vi "Instantiate.vi"(0 "scripts manager in":refnum<class "scripts manager.lvclass">, 5 "Output Terminal":refnum<class "Output Terminal.lvclass">, 7 "RT Variables":refnum<class "RT Variables.lvclass">, 9 "Function Directory[]":path[](array[path]), 11 "error in (no error)":errorcluster) -> (4 "scripts manager out":refnum<class "scripts manager.lvclass">, 15 "error out":errorcluster)   [LabVIEW 2019, in "LSL.lvlib" / "scripts manager.lvclass"]
uses:
  scripts manager.lvclass
  output terminal/Base/Output Terminal.lvclass
  variables/RT Variables/RT Variables.lvclass
  scripts manager.lvclass/scripts manager.ctl
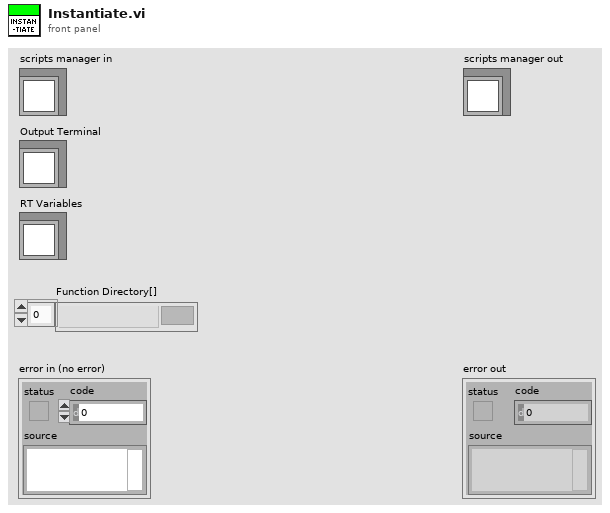
[diagram p1: front panel]
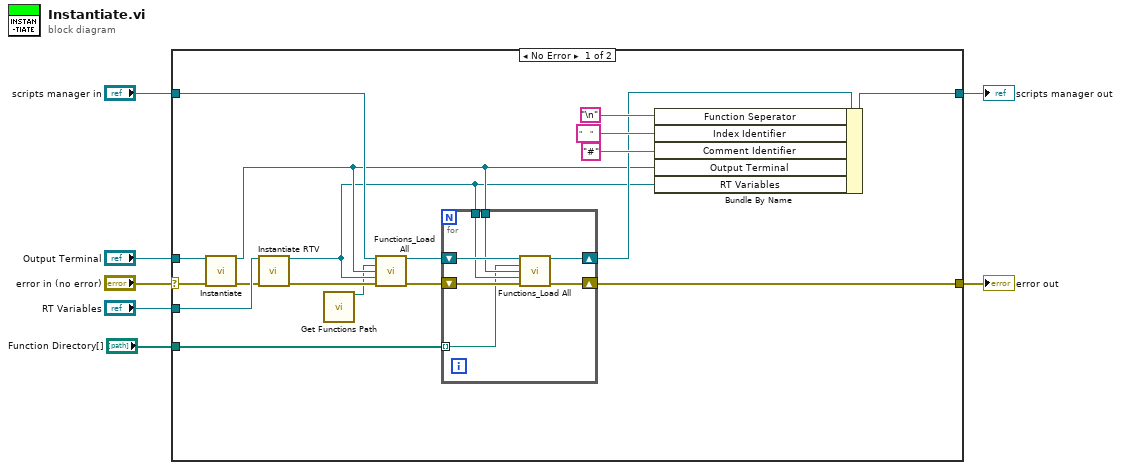
[diagram p0: block diagram]
diagram:
  n1 = case shown="No Error" "error in (no error)" {
    selector: "error in (no error)" -> [w17 w34]
    tunnel: [w14 w34] -> w6
    tunnel: [w25 w33] -> w4
    tunnel: "scripts manager in" -> [w21 w33]
    tunnel: "Output Terminal" -> [w18 _]
    tunnel: "RT Variables" -> [w19 _]
    tunnel: "Function Directory[]" -> [w8 _]
    frame No Error {
      n2 = call-dynamic "Instantiate.vi"("Output Terminal in"=w18, "error in (no error)"=w17) -> ("Output Terminal out"=w11:refnum<class "Output Terminal.lvclass">, "error out"=w16:errorcluster)  [unwired: 12 in]
      n3 = call-dynamic "Instantiate RTV.vi"("RT Variables in"=w19, "error in (no error)"=w16) -> ("RT Variables out"=w10:refnum<class "RT Variables.lvclass">, "error out"=w20:errorcluster)  [unwired: 12 in]
      n4 = call "Get Functions Path.vi"() -> ("Basic Function List"=w9:path)  [unwired: 13 in, 2 out]
      n5 = call-dynamic "Functions_Load All.vi"("scripts manager in"=w21, "Function Path"=w9, "Output Terminal"=w11, "RT Variables"=w10, "error in (no error)"=w20) -> ("scripts manager out"=w13:refnum<class "scripts manager.lvclass">, "error out"=w15:errorcluster)  [unwired: 9 in]
      n6 = for {
        tunnel: w11 -> [w28]
        tunnel: w10 -> [w27]
        shift-right: [w31] -> w14
        shift-left: w15 -> [w32]
        shift-right: [w29] -> w12
        shift-left: w13 -> [w30]
        tunnel: w8 -> [w26] mode=indexing
        n7 = call-dynamic "Functions_Load All.vi"("scripts manager in"=w30, "Function Path"=w26, "Output Terminal"=w28, "RT Variables"=w27, "error in (no error)"=w32) -> ("scripts manager out"=w29:refnum<class "scripts manager.lvclass">, "error out"=w31:errorcluster)  [unwired: 9 in]
      }
      n8 = Bundle By Name(cluster=w12, "Function Seperator"="\n", "Index Identifier"="    " ("Function Rules.Index Identifier"), "Comment Identifier"="#" ("Function Rules.Comment Identifier"), "Output Terminal"=w11, "RT Variables"=w10) -> (w25:refnum<class "scripts manager.lvclass">)
    }
    frame Error {
    }
  }
  "error out" <- w6
  "scripts manager out" <- w4
